vi "add-br-.vi"() -> ()   [LabVIEW 2018]
panel:
  out "result string":string
  out "x = y?":bool
  out "concatenated string":string
  out "text":string
  in  "file (use dialog)":path
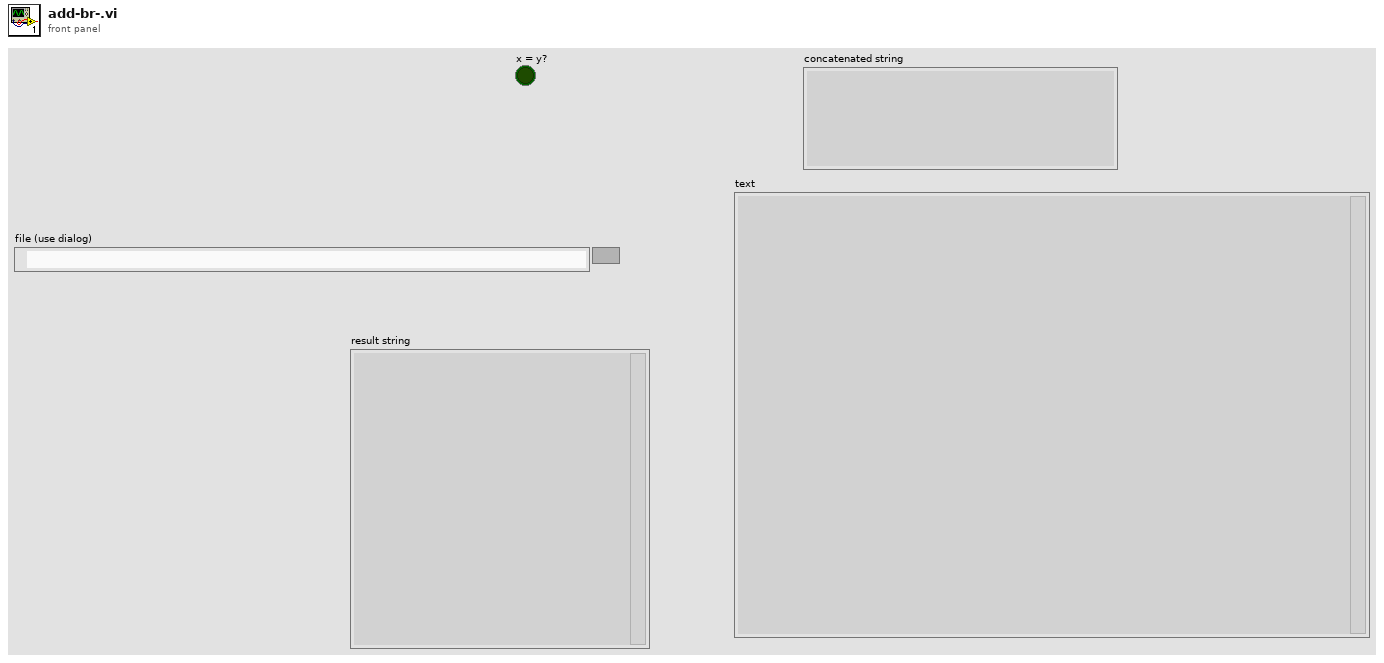
[diagram p1: front panel]
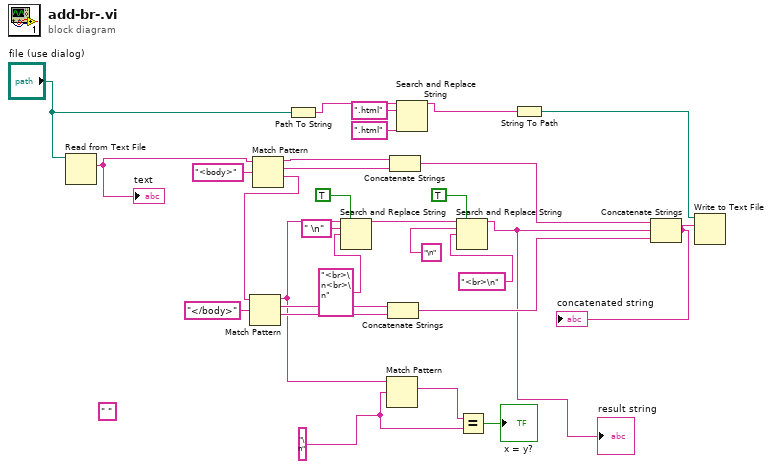
[diagram p0: block diagram]
diagram:
  (unwired) " " ("search string")
  w7 = "\n" ("search string")
  n1 = Read from Text File(file (use dialog)="file (use dialog)") -> (text=w29:string)  [unwired: 3 in, 3 out]
  "text" <- w29
  n2 = Match Pattern(string=w29, regular expression="<body>") -> (before substring=w25:string, match substring=w24:string, after substring=w19:string)  [unwired: 1 in, 1 out]
  n3 = Match Pattern(string=w19, regular expression="</body>") -> (before substring=w5:string, match substring=w23:string, after substring=w22:string)  [unwired: 1 in, 1 out]
  n4 = Path To String(path="file (use dialog)") -> (string=w14:string)
  n5 = Search and Replace String(replace all?=TRUE ("replace all? (F)"), input string=w5, search string=" \n", replace string="<br>\n<br>\n" ("replace string (\"\")")) -> (result string=w4:string)  [unwired: 4 in, 3 out]
  n6 = Match Pattern(string=w5, regular expression=w7) -> (match substring=w8:string)  [unwired: 1 in, 3 out]
  n7 = Concatenate Strings(w23, w22) -> (w20:string)
  n8 = Concatenate Strings(w25, w24) -> (w21:string)
  n9 = Search and Replace String(input string=w14, search string=".html", replace string=".html" ("replace string (\"\")")) -> (result string=w13:string)  [unwired: 5 in, 3 out]
  n10 = Search and Replace String(replace all?=TRUE ("replace all? (F)"), input string=w4, search string="\n", replace string="<br>\n" ("replace string (\"\")")) -> (result string=w16:string)  [unwired: 4 in, 3 out]
  "result string" <- w16
  n11 = Equal?(x=w8, y=w7) -> (x = y?=→"x = y?":bool)
  n12 = String To Path(string=w13) -> (path=w10:path)
  n13 = Concatenate Strings(w21, w16, w20) -> (w15:string)
  "concatenated string" <- w15
  n14 = Write to Text File(file (use dialog)=w10, text=w15) -> ()  [unwired: 2 in, 3 out]
